vi "setDeviceNameToDevice.vi"(0 "Controller in":refnum<class "_Controller.lvclass">, 2 "device_name (in)":string, 5 "error in (no error)":errorcluster) -> (14 "Controller out":refnum<class "_Controller.lvclass">, 17 "success?":bool, 18 "response":string, 19 "error out":errorcluster)   [LabVIEW 2020, in "classes.lvlib" / "_Controller.lvclass"]
doc: "Sets the specified Device Name to the referenced device\n\nProduced By:\n\n<B>Kod Integrations, LLC</B>\n4835 Marianne Drive\nMount Airy, MD 21771\nhttp://www.kodintegrations.com\nemail: info@kodintegrations.com\nphone: (240) 687-1288"
uses:
  _Controller.lvclass
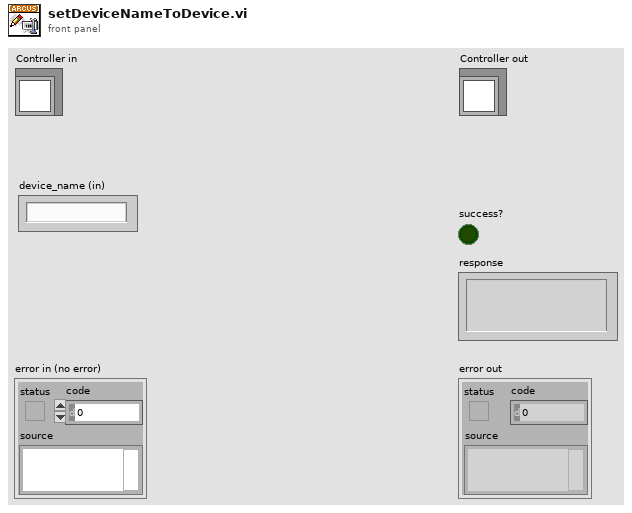
[diagram p1: front panel]
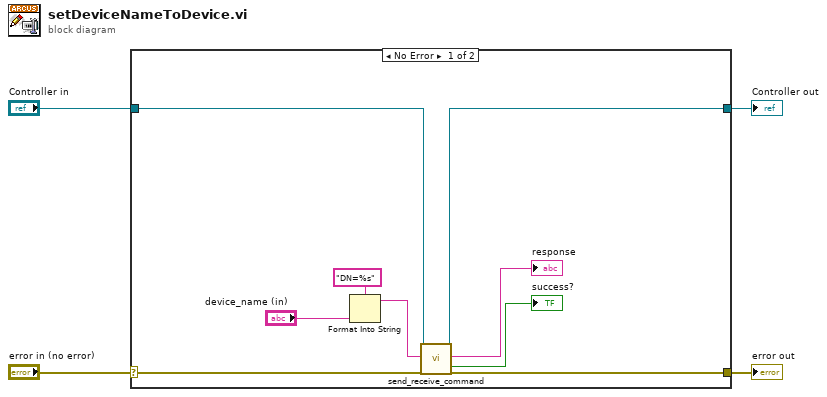
[diagram p0: block diagram]
diagram:
  n1 = case shown="No Error" "error in (no error)" {
    selector: "error in (no error)" -> [w13 w15]
    tunnel: [w12 w15] -> w3
    tunnel: [w8 w14] -> w1
    tunnel: "Controller in" -> [w9 w14]
    frame No Error {
      n2 = Format Into String(format string="DN=%s", "device_name (in)") -> (resulting string=w5:string)  [unwired: 2 in, 1 out]
      n3 = call "send_receive_command.vi"("reference (in)"=w9, "ASCII Command (in)"=w5, "error in (no error)"=w13) -> ("reference (out)"=w8:refnum<class "_Controller.lvclass">, "response (out)"=→"response":string, "success?"=→"success?":bool, "error out"=w12:errorcluster)  [unwired: 12 in, 1 out]
    }
    frame Error {
    }
  }
  "error out" <- w3
  "Controller out" <- w1
